vi "Autonomous Independent.vi"() -> ()   [LabVIEW 2018]
doc: "This VI is called when autonomous begins, and will automatically be terminated when autonomous ends. You can carry out timed or sensor driven robot movement independently without needing to return to the caller."
uses:
  Drivebase/Drive Motion Magic Setpoints.ctl
  <vilib>/Rock Robotics/Network Tables/NT Read String.vi
  Robot Global Data.vi
  <vilib>/Rock Robotics/Network Tables/NT Write Number.vi
  <vilib>/Rock Robotics/WPI/Utilities/WPI_GetSetVariantRefNum.vi
  <vilib>/Rock Robotics/Network Tables/NT Write Boolean Array.vi
  <vilib>/Rock Robotics/Network Tables/NT Write Numeric Array.vi
panel:
  in  "Array of robot movements":T1(array[cluster])=[{"X Joystick Value"=0.39393939393939403, "Y Joystick Value"=0.0, "Delay (sec)"=1.0, "Movement Name"="turn"}, {"X Joystick Value"=-0.3737373737373737, "Y Joystick Value"=0.0, "Delay (sec)"=1.0, "Movement Name"="turn back"}] {"Y Joystick Value" scale=1.0..-1.0; "X Joystick Value" scale=-1.0..1.0}
  # "Be sure to right-click and choose Data Operations>>Make Current Value default if you want to save the array values with the VI"
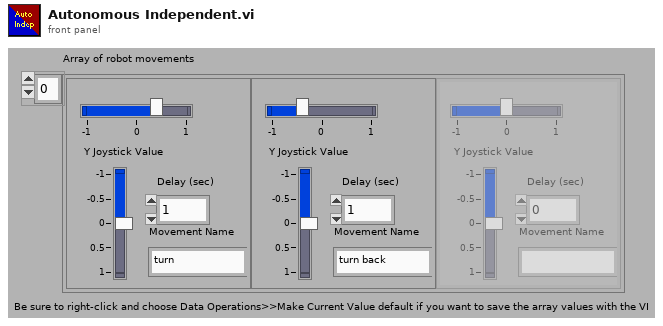
[diagram p1: front panel]
types:
  T1 = cluster{"X Joystick Value":dbl, "Y Joystick Value":dbl, "Delay (sec)":dbl, "Movement Name":string}[]
  T2 = typedef "Auton Movements.ctl" = cluster{"Drive":dbl, "TurnDegrees":dbl, "4bar state":T3}
  T3 = typedef "4bar state enum.ctl" = enum16{"High", "Middle", "Low", "Ground"}
  T4 = typedef "Drive Motion Magic Setpoints.ctl" = cluster{"Increase in Left":dbl, "Increase in Right":dbl}
  T5 = typedef "WPI_JoystickDevRef.ctl" = cluster{"Device":T6}
  T6 = typedef "WPI_JoystickDeviceEnum.ctl" = enum16{"USB 0", "USB 1", "USB 2", "USB 3", "USB 4", "USB 5"}
  T7 = typedef "Joystick Controls.ctl" = cluster{"Driver Left Joystick X":dbl, "Driver Left Joystick Y":dbl, "Driver A Button":bool, "Driver B Button":bool, "Driver X Button":bool, "Driver Y Button":bool, "Driver Left Bumper":bool, "Driver Right Bumper":bool, "Driver View Button":bool, "Driver Menu Button":bool, "Driver Left Joystick Press":bool, "Driver Right Joystick Press":bool, "Driver Left Trigger":dbl, "Driver Right Joystick X":dbl, "Driver Right Joystick Y":dbl, "Driver Right Trigger":dbl, "Operator Left Joystick X":dbl, "Operator Left Joystick Y":dbl, "Operator A Button":bool, "Operator B Button":bool, "Operator X Button":bool, "Operator Y Button":bool, "Operator Left Bumper":bool, "Operator Right Bumper":bool, "Operator View Button":bool, "Operator Menu Button":bool, "Operator Left Joystick Press":bool, "Operator Right Joystick Press":bool, "Operator Left Trigger":dbl, "Operator Right Joystick X":dbl, "Operator Right Joystick Y":dbl, "Operator Right Trigger":dbl, "Driver D-Pad":i16, "Operator D-Pad":i16}
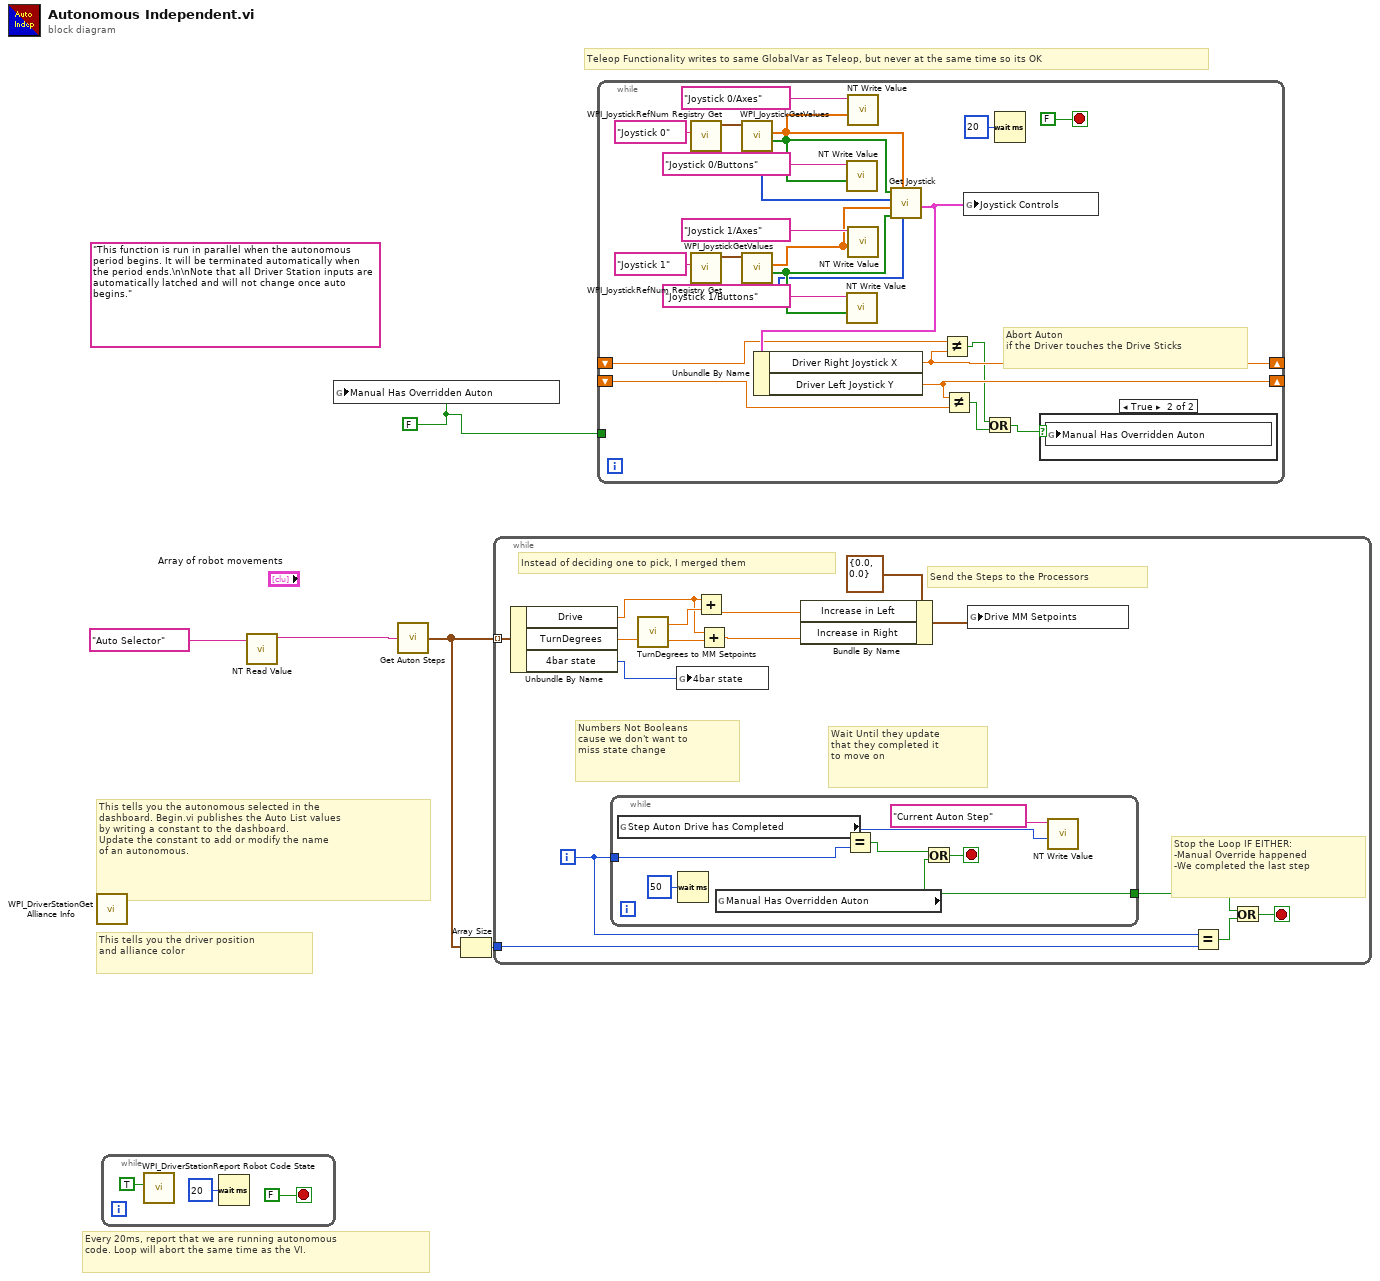
[diagram p0: block diagram]
diagram:
  w2 = FALSE
  (unwired) "This function is run in parallel when the autonomous period begins. It will be terminated automatically when the period ends.\n\nNote that all Driver Station inputs are automatically latched and will not change once auto begins."
  # "Teleop Functionality writes to same GlobalVar as Teleop, but never at the same time so its OK"
  # "This tells you the autonomous selected in the \ndashboard. Begin.vi publishes the Auto List values\nby writing a constant to the dashboard.\nUpdate the constant to add or modify the name\nof an autonomous."
  # "Every 20ms, report that we are running autonomous\ncode. Loop will abort the same time as the VI."
  # "This tells you the driver position\nand alliance color"
  n1 = call <vilib>:"WPI_DriverStationGet Alliance Info.vi"() -> ()  [unwired: 12 out]
  n2 = while {
    stop <- FALSE stop-if-true
    n3 = call <vilib>:"WPI_DriverStationReport Robot Code State.vi"("Autonomous"=TRUE) -> ()  [unwired: 10 in, 1 out]
    n4 = Wait (ms)(milliseconds to wait=u32 20) -> ()  [unwired: 1 out]
  }
  n5 = call-poly <vilib>:"NT Read Value.vi"("Name"="Auto Selector") -> ("String"=w4:string)  [unwired: 9 in, 1 out]
  n6 = global write "Robot Global Data.vi" "Manual Has Overridden Auton"(w2) -> ()
  n7 = call "Get Auton Steps.vi"("Name of Auton to Do"=w4) -> ("Output Movements"=w1:T2[])
  n8 = Array Size(array=w1) -> (size(s)=w3:i32)
  n9 = while {
    tunnel: w3 -> [w19]
    tunnel: w1 -> [w12] mode=indexing
    i -> [w20]
    stop <- w21 stop-if-true
    # "Instead of deciding one to pick, I merged them"
    # "Stop the Loop IF EITHER: \n-Manual Override happened\n-We completed the last step"
    # "Numbers Not Booleans \ncause we don't want to \nmiss state change"
    # "Wait Until they update \nthat they completed it \nto move on"
    # "Send the Steps to the Processors"
    n10 = Unbundle By Name(w12) -> ("Drive"=w11:dbl, "TurnDegrees"=w10:dbl, "4bar state"=w9:T3)
    n11 = while {
      tunnel: w20 -> [w30]
      tunnel: [w24] -> w23
      stop <- w27 stop-if-true
      n12 = global read "Robot Global Data.vi" "Step Auton Drive has Completed"() -> (w25:i32)
      n13 = Wait (ms)(milliseconds to wait=u32 50) -> ()  [unwired: 1 out]
      n14 = global read "Robot Global Data.vi" "Manual Has Overridden Auton"() -> (w24:bool)
      n15 = Equal?(x=w25, y=w30) -> (x = y?=w28:bool)
      n16 = Or(x=w28, y=w24) -> (x .or. y?=w27:bool)
      n17 = call-poly <vilib>:"NT Write Value.vi"("Numeric"=w25, "Name"="Current Auton Step") -> ()  [unwired: 9 in, 1 out]
    }
    n18 = call "TurnDegrees to MM Setpoints.vi"("Turn Degrees"=w10) -> ("Right MM Setpoint"=w13:dbl, "Left MM Setpoint"=w15:dbl)  [unwired: 1 in]
    n19 = global write "Robot Global Data.vi" "4bar state"(w9) -> ()
    n20 = Add(x=w11, y=w15) -> (x+y=w16:dbl)
    n21 = Add(x=w11, y=w13) -> (x+y=w14:dbl)
    n22 = Bundle By Name(cluster=T4 {"Increase in Left"=0.0, "Increase in Right"=0.0} ("Drive MM Setpoints"), "Increase in Left"=w16, "Increase in Right"=w14) -> (w18:T4)
    n23 = global write "Robot Global Data.vi" "Drive MM Setpoints"(w18) -> ()
    n24 = Equal?(x=w20, y=w19) -> (x = y?=w22:bool)
    n25 = Or(x=w23, y=w22) -> (x .or. y?=w21:bool)
  }
  n26 = while {
    shift-right: [w35] -> _
    shift-left: _ -> [w34]
    shift-right: [w36] -> _
    shift-left: _ -> [w37]
    tunnel: w2 -> [_]
    stop <- FALSE stop-if-true
    # "Abort Auton\nif the Driver touches the Drive Sticks"
    n27 = call <vilib>:"WPI_JoystickRefNum Registry Get.vi"("refnum name"="Joystick 0") -> ("JoystickDevRef"=w52:T5)  [unwired: 1 in, 9 out]
    n28 = call <vilib>:"WPI_JoystickRefNum Registry Get.vi"("refnum name"="Joystick 1") -> ("JoystickDevRef"=w49:T5)  [unwired: 1 in, 9 out]
    n29 = call <vilib>:"WPI_JoystickGetValues.vi"("JoystickDevRef"=w52) -> ("Buttons"=w45:bool[], "Axes"=w44:dbl[], "POVs"=w43:i16[])  [unwired: 6 in, 2 out]
    n30 = call <vilib>:"WPI_JoystickGetValues.vi"("JoystickDevRef"=w49) -> ("Buttons"=w41:bool[], "Axes"=w42:dbl[], "POVs"=w40:i16[])  [unwired: 6 in, 2 out]
    n31 = call-poly <vilib>:"NT Write Value.vi"("Boolean Array"=w45, "Name"="Joystick 0/Buttons") -> ()  [unwired: 9 in, 1 out]
    n32 = call-poly <vilib>:"NT Write Value.vi"("Boolean Array"=w41, "Name"="Joystick 1/Buttons") -> ()  [unwired: 9 in, 1 out]
    n33 = call-poly <vilib>:"NT Write Value.vi"("Numeric Array"=w44, "Name"="Joystick 0/Axes") -> ()  [unwired: 9 in, 1 out]
    n34 = call-poly <vilib>:"NT Write Value.vi"("Numeric Array"=w42, "Name"="Joystick 1/Axes") -> ()  [unwired: 9 in, 1 out]
    n35 = call "Get Joystick.vi"("Operator POVs"=w40, "Driver Axes"=w44, "Operator Buttons"=w41, "Operator Axes"=w42, "Driver POVs"=w43, "Driver Buttons"=w45) -> ("Joystick Controls Out"=w38:T7)
    n36 = Unbundle By Name(w38) -> ("Driver Right Joystick X"=w36:dbl, "Driver Left Joystick Y"=w35:dbl)
    n37 = Not Equal?(x=w37, y=w36) -> (x != y?=w33:bool)
    n38 = Not Equal?(x=w35, y=w34) -> (x != y?=w32:bool)
    n39 = global write "Robot Global Data.vi" "Joystick Controls"(w38) -> ()
    n40 = Or(x=w33, y=w32) -> (x .or. y?=w31:bool)
    n41 = Wait (ms)(milliseconds to wait=u32 20) -> ()  [unwired: 1 out]
    n42 = case shown="True" w31 {
      selector: w31 -> [_ w55]
      frame False {
      }
      frame True {
        n43 = global write "Robot Global Data.vi" "Manual Has Overridden Auton"(w55) -> ()
      }
    }
  }
